vi "MeasureProcess_FGV.vi"(0 "write status":T1, 1 "action":T3(ring), 5 "ProjectAct step":T2(ring), 11 "error in":errorcluster, 12 "new element/subarray":string) -> (4 "read project name":string, 6 "read project step":string[](array[string]), 8 "step content":string[](array[string]), 10 "Table Control":string[][](table), 15 "error out":errorcluster)   [LabVIEW 2019]
uses:
  Ctrl/ProjectNameSelect.ctl
  e17d802b-cf53-46b2-bed7-7df0a5bdc549.vi
  <vilib>/JDP Science/JSONtext/Variant to JSON Text.vi
  fab65405-55d6-4226-9659-8694a5ed6800.vi
  LLB/Commonly VI/Main Glb.vi
  LLB/Commonly VI.lvlib
  <vilib>/drjdpowell/SQLite Library/SQL Connection/Execute SQL (Single String).vi
panel:
  out "element":string
  in  "Project Index":i32=3
  # "Up:0\nDown:1"
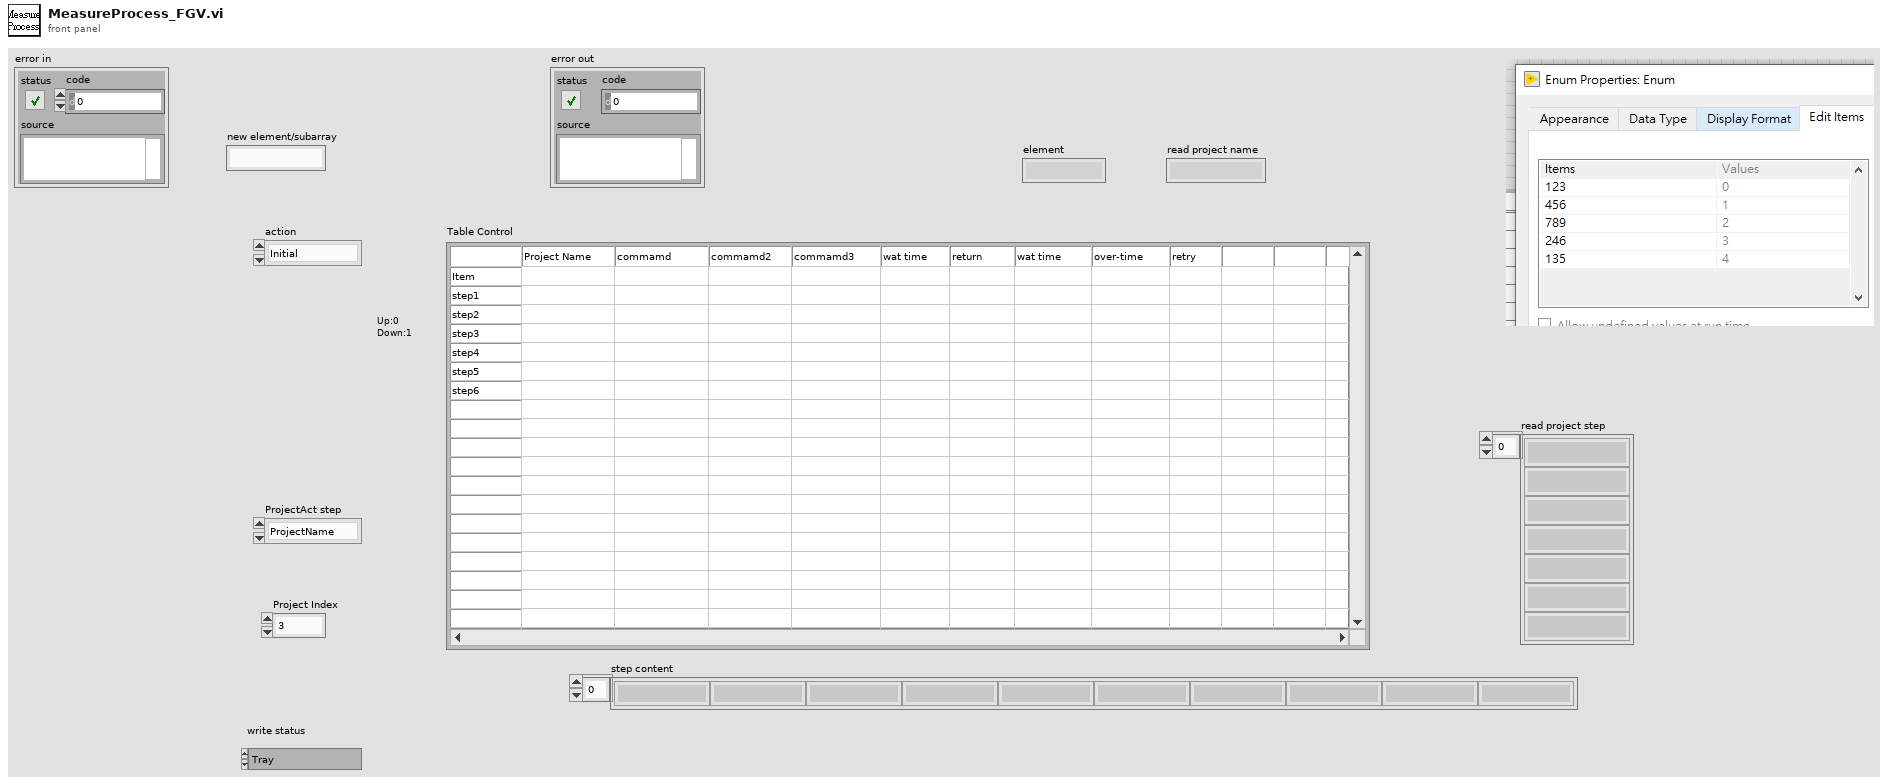
[diagram p1: front panel]
types:
  T1 = typedef "ProjectNameSelect.ctl" = enum16{"Tray", "NewItem", "NoTray", "Working", "OK"}
  T2 = enum16{"ProjectName", "Name", "Initial", "Reset", "Format", "Program1", "Program2", "Scan"}
  T3 = enum16{"Initial", "load", "read", "write", "write sn", "save"}
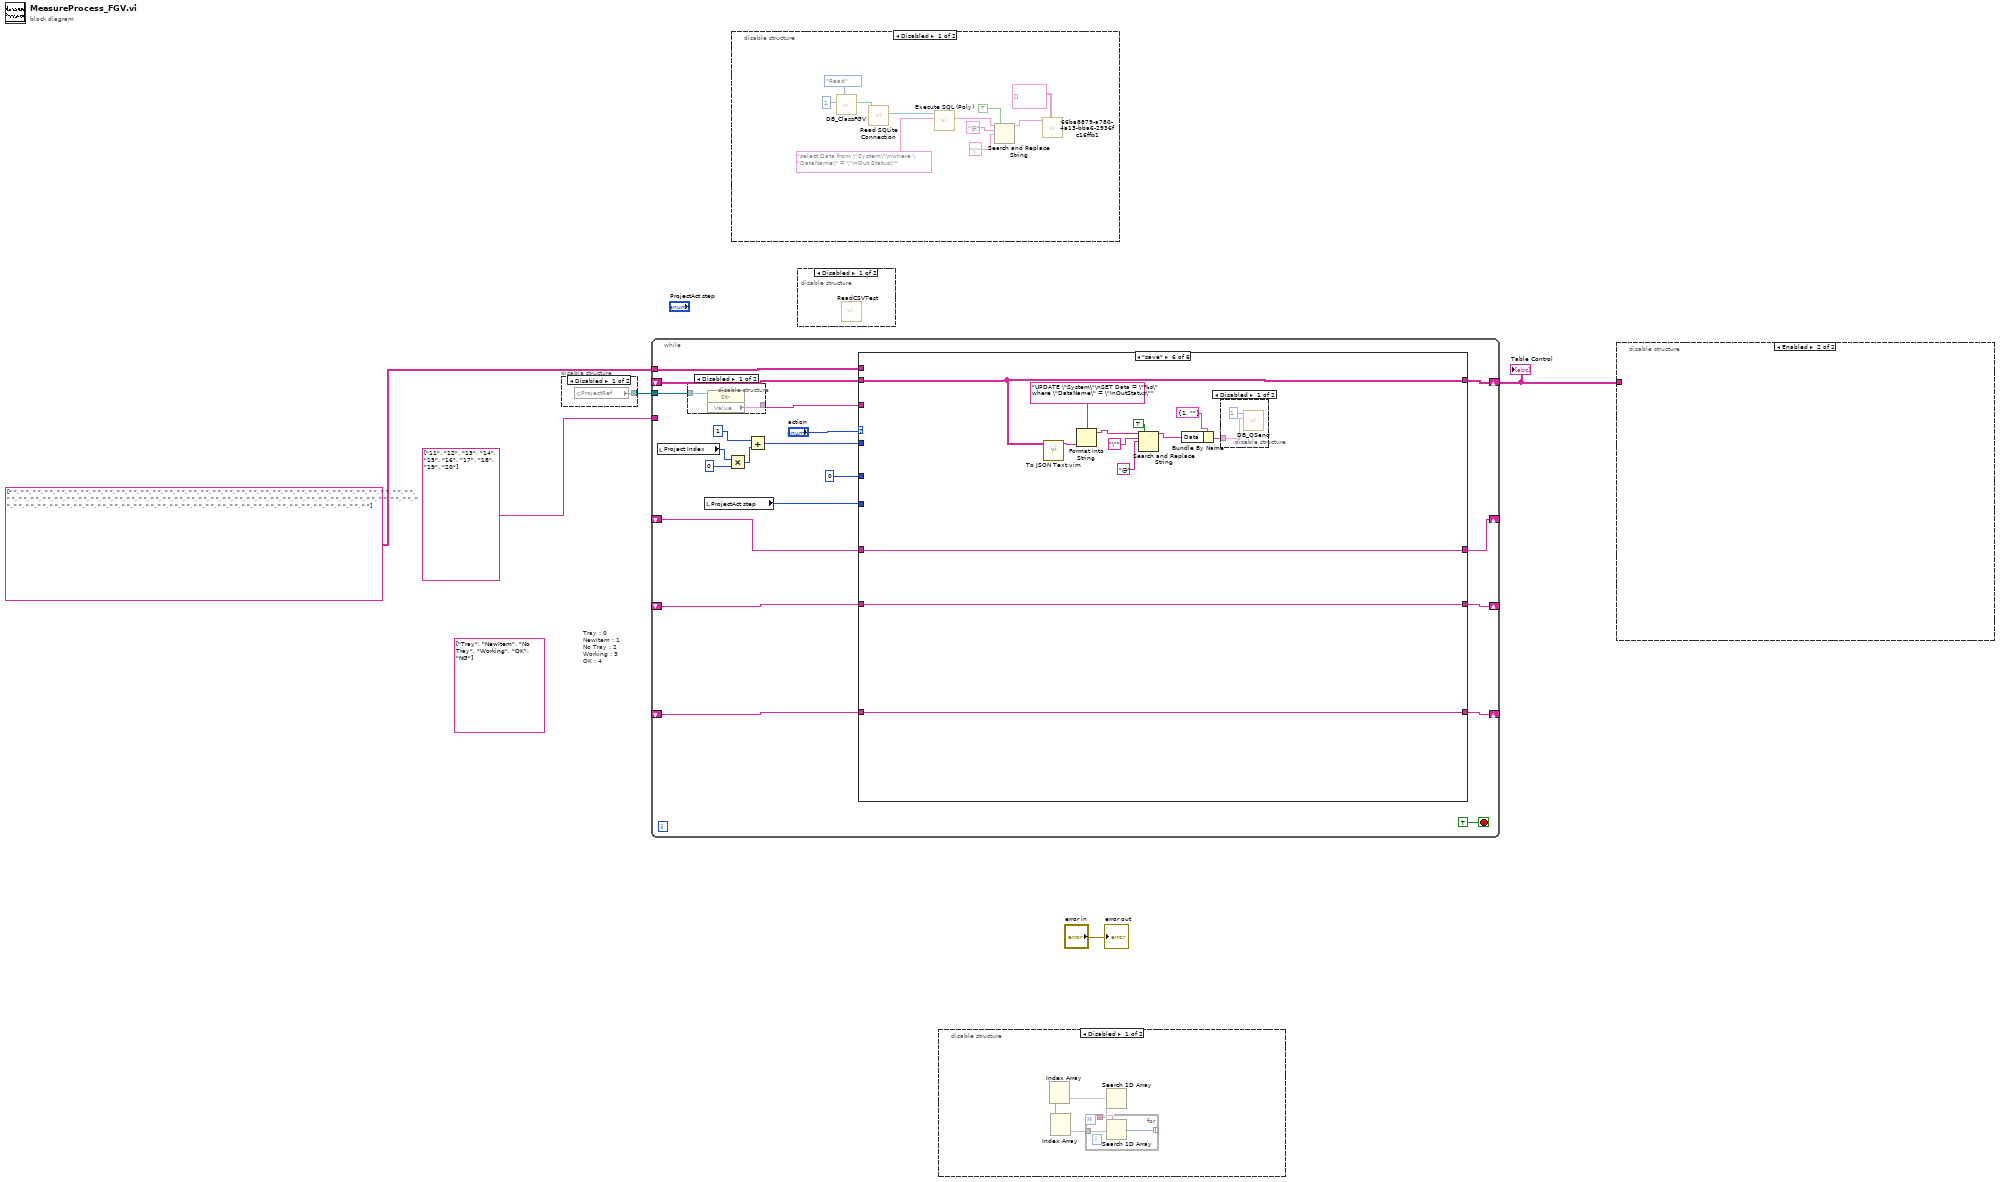
[diagram p0: block diagram]
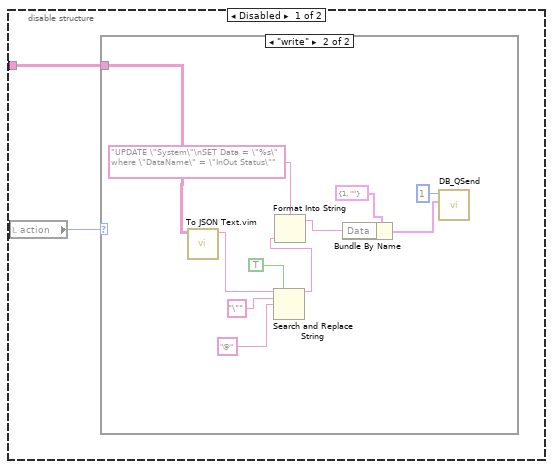
[diagram p6: hidden frame]
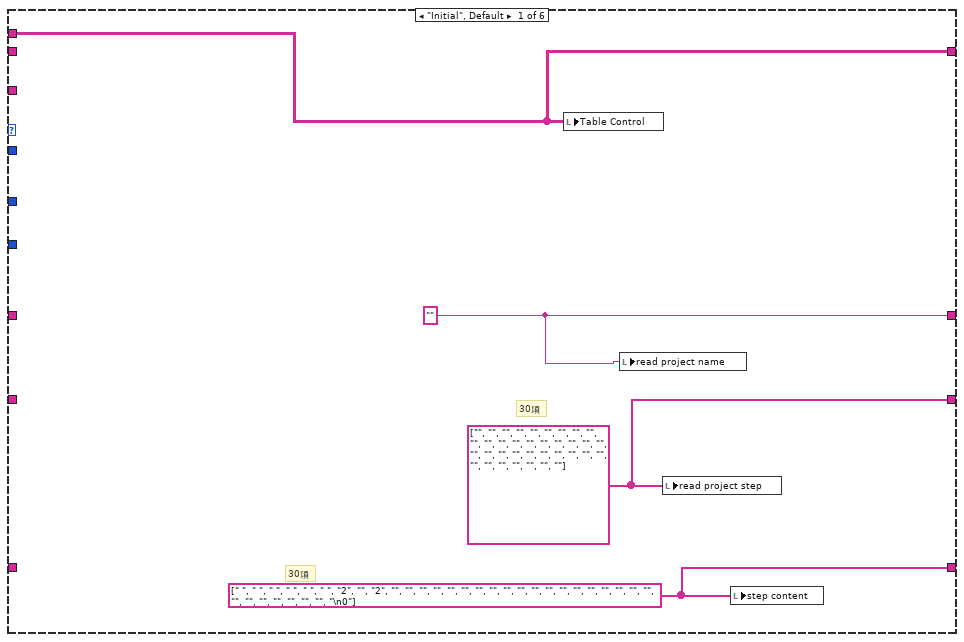
[diagram p9: hidden frame]
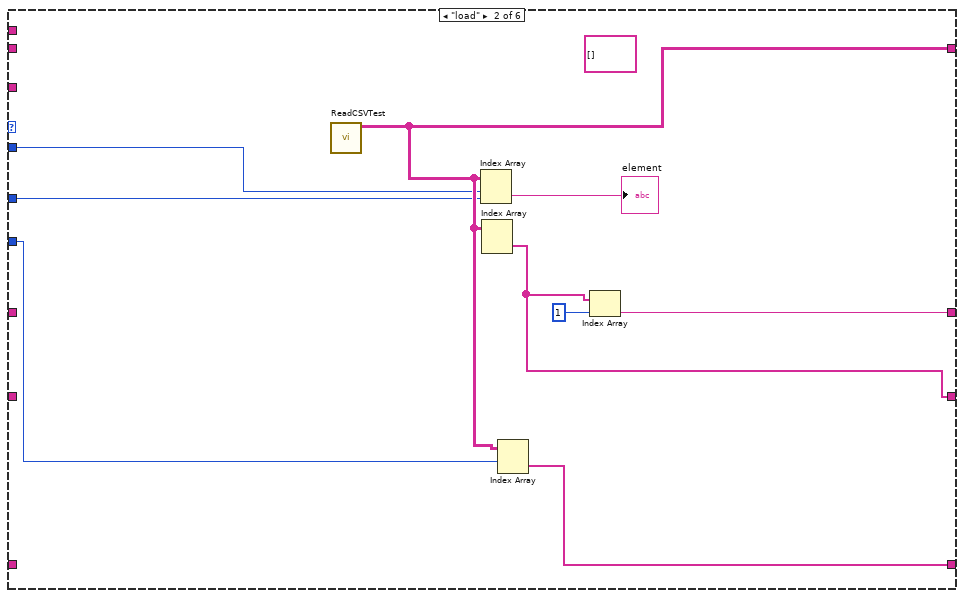
[diagram p10: hidden frame]
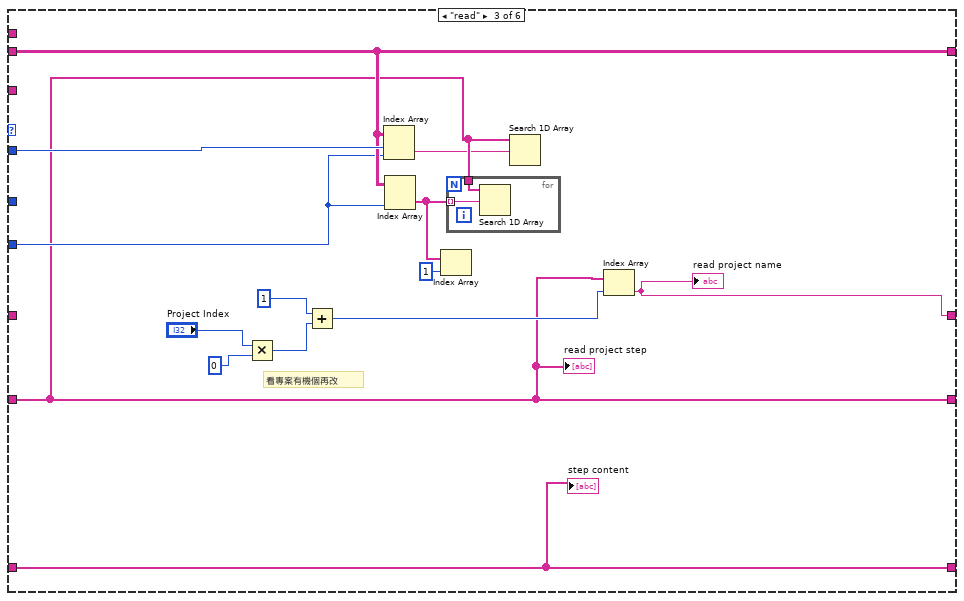
[diagram p11: hidden frame]
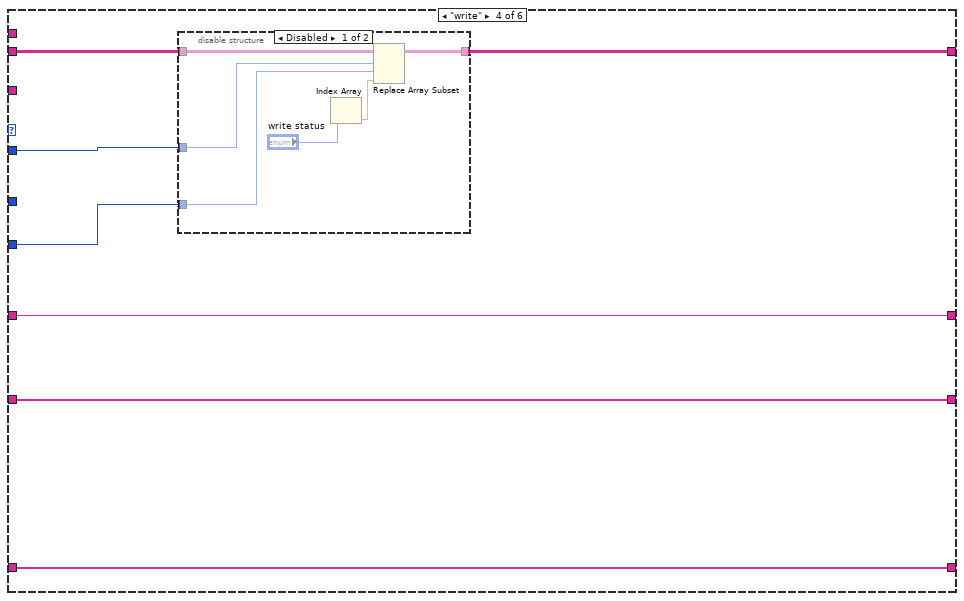
[diagram p12: hidden frame]
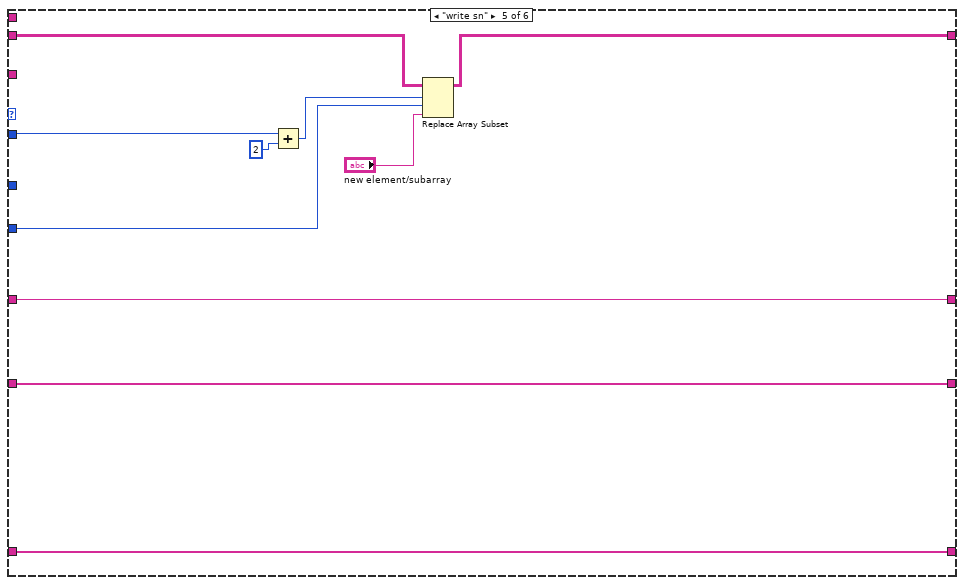
[diagram p14: hidden frame]
diagram:
  (unwired) string[] ["Tray", "NewItem", "No Tray", "Working", "OK", "NG"]
  # "Tray : 0\nNewItem : 1\nNo Tray : 2\nWorking : 3\nOK : 4"
  n1 = disable-structure shown="Disabled" {
    disable-tunnel: [w6 _] -> w2
    frame Disabled {
      n2 = global read "Main Glb.vi" "ProjectRef"() -> (w6:refnum<vi>)
    }
    frame Enabled {
    }
  }
  n3 = while {
    shift-right: [w24] -> w4
    shift-left: _ -> [w23]
    tunnel: string[] ["11", "12", "13", "14", "15", "16", "17", "18", "19", "20"] -> [_]
    shift-right: [w22] -> _
    shift-left: _ -> [w18]
    shift-right: [w21] -> _
    shift-left: _ -> [w17]
    shift-right: [w20] -> _
    shift-left: _ -> [w19]
    tunnel: w2 -> [w10]
    tunnel: string[][] [[" ", " ", " ", " ", " ", " ", " ", " ", " ", " ", " "], [" ", " ", " ", " ", " ", " ", " ", " ", " ", " ", " "], [" ", " ", " ", " ", " ", " ", " ", " ", " ", " ", " "], [" ", " ", " ", " ", " ", " ", " ", " ", " ", " ", " "], [" ", " ", " ", " ", " ", " ", " ", " ", " ", " ", " "], [" ", " ", " ", " ", " ", " ", " ", " ", " ", " ", " "], [" ", " ", " ", " ", " ", " ", " ", " ", " ", " ", " "], [" ", " ", " ", " ", " ", " ", " ", " ", " ", " ", " "], [" ", " ", " ", " ", " ", " ", " ", " ", " ", " ", " "]] -> [w7]
    stop <- TRUE stop-if-true
    n4 = local read "Project Index"() -> (w14:i32)
    n5 = disable-structure shown="Disabled" {
      disable-tunnel: w10 -> [w28 _]
      disable-tunnel: [w27 _] -> w9
      frame Disabled {
        n6 = property class="Str"(reference=w28) -> ("Value"=w27:string)  [unwired: 1 in, 2 out]
      }
      frame Enabled {
      }
    }
    n7 = local read "ProjectAct step"() -> (w16:T2)
    n8 = Multiply(x=w14, y=0) -> (x*y=w15:i32)
    n9 = Add(x=1, y=w15) -> (x+y=w11:i32)
    n10 = case shown="\"save\"" "action" {
      tunnel: [w29 w41 w54 w63 w79 w85] -> w24
      tunnel: w23 -> [_ _ w54 w64 w80 w85]
      tunnel: w16 -> [_ w33 w50 w62 w78 _]
      tunnel: w11 -> [_ w40 w55 w61 w76 _]
      tunnel: [w32 w36 w49 w60 w73 w83] -> w22
      tunnel: [w31 w37 w43 w59 w72 w82] -> w21
      tunnel: [w30 w39 w53 w58 w71 w81] -> w20
      tunnel: w19 -> [_ _ w53 w58 w71 w81]
      tunnel: w18 -> [_ _ _ w60 w73 w83]
      tunnel: w17 -> [_ _ w43 w59 w72 w82]
      tunnel: w9 -> [_ _ _ _ _ _]
      tunnel: 0 -> [_ w34 _ _ _ _]
      tunnel: w7 -> [w29 _ _ _ _ _]
      frame "Initial", Default {
        w30 = string[] [" ", " ", " ", " ", " ", " ", "2", "", "2", "", "", "", "", "", "", "", "", "", "", "", "", "", "", "", "", "", "", "", "", "", "", "", "", "", "", "\n0"] ("step content")
        w31 = string[] ["", "", "", "", "", "", "", "", "", "", "", "", "", "", "", "", "", "", "", "", "", "", "", "", "", "", "", "", "", "", "", "", "", "", "", ""] ("read project step")
        w32 = "" ("String")
        # "30項"
        # "30項"
        n11 = local write "Table Control"(w29) -> ()
        n12 = local write "read project name"(w32) -> ()
        n13 = local write "read project step"(w31) -> ()
        n14 = local write "step content"(w30) -> ()
      }
      frame "load" {
        (unwired) string[][] [] ("Table Control")
        n15 = call "ReadCSVTest.vi"() -> ("all rows"=w41:string[][])  [unwired: 11 in]
        n16 = Index Array(array=w41, index (row)=w40, index (col)=w34) -> (element=→"element":string)
        n17 = Index Array(array=w41) -> (element=w37:string[])  [unwired: 2 in]
        n18 = Index Array(array=w41, index (row)=w33) -> (element=w39:string[])  [unwired: 1 in]
        n19 = Index Array(array=w37, index=1) -> (element=w36:string)
      }
      frame "read" {
        # "看專案有機個再改"
        n20 = Multiply(x="Project Index", y=0) -> (x*y=w44:i32)
        n21 = Add(x=1, y=w44) -> (x+y=w47:i32)
        n22 = Index Array(array=w54, index (row)=w55, index (col)=w50) -> (element=w42:string)
        n23 = Index Array(array=w54, index (col)=w50) -> (element=w51:string[])  [unwired: 1 in]
        n24 = Index Array(array=w51, index=1) -> ()  [unwired: 1 out]
        n25 = for {
          tunnel: w43 -> [w57]
          tunnel: w51 -> [w56] mode=indexing
          n26 = Search 1D Array(1D array=w57, element=w56) -> ()  [unwired: 1 in, 1 out]
        }
        n27 = Search 1D Array(1D array=w43, element=w42) -> ()  [unwired: 1 in, 1 out]
        n28 = Index Array(array=w43, index=w47) -> (element=w49:string)
        "read project name" <- w49
        "read project step" <- w43
        "step content" <- w53
      }
      frame "write" {
        n29 = disable-structure shown="Disabled" {
          disable-tunnel: w64 -> [w70 _]
          disable-tunnel: [w69 _] -> w63
          disable-tunnel: w62 -> [w66 _]
          disable-tunnel: w61 -> [w65 _]
          frame Disabled {
            n30 = Index Array(index="write status") -> (element=w68)  [unwired: 1 in]
            n31 = Replace Array Subset(array=w70, new element=w68, index (row)=w65, index (col)=w66) -> (w69:string[][])
          }
          frame Enabled {
          }
        }
      }
      frame "write sn" {
        n32 = Add(x=w76, y=2) -> (x+y=w77:i32)
        n33 = Replace Array Subset(array=w80, new element="new element/subarray", index (row)=w77, index (col)=w78) -> (w79:string[][])
      }
      frame "save" {
        n34 = call "To JSON Text.vim"("Anything"=w85) -> ("<JSON>"=w91:string)  [unwired: 9 in, 1 out]
        n35 = Format Into String(format string="UPDATE \"System\"\nSET Data = \"%s\" where \"DataName\" = \"InOutStatus\"", w91) -> (resulting string=w87:string)  [unwired: 2 in, 1 out]
        n36 = Search and Replace String(replace all?=TRUE ("replace all? (F)"), input string=w87, search string="\"", replace string="@" ("replace string (\"\")")) -> (result string=w86:string)  [unwired: 4 in, 3 out]
        n37 = Bundle By Name(cluster=cluster{"Record":i32, "Data":string} {"Record"=1, "Data"=""} ("Data"), "Data"=w86) -> (w90:cluster{"Record":i32, "Data":string})
        n38 = disable-structure shown="Disabled" {
          disable-tunnel: w90 -> [w94 _]
          frame Disabled {
            n39 = call "DB_QSend.vi"("Data"=w94, "Threadindex"=1) -> ()  [unwired: 9 in, 1 out]
          }
          frame Enabled {
          }
        }
      }
    }
  }
  "Table Control" <- w4
  n40 = disable-structure shown="Disabled" {
    frame Disabled {
      n41 = call "DB_ClassFGV.vi"("Enum"=enum16{"initial", "Write", "Read"}."Read", "index"=1) -> ("DB Class out"=w98:refnum<class "DataBase.lvclass">)  [unwired: 7 in, 2 out]
      n42 = call-dynamic "Read SQLite Connection.vi"("DataBase in"=w98) -> ("SQLite.lvlib:Connection"=w99:refnum<class "Connection.lvclass">)  [unwired: 8 in, 2 out]
      n43 = call-poly <vilib>:"Execute SQL (Poly).vi"("SQL"="select Data from \"System\"\nwhere \"DataName\" = \"InOut Status\"", "SQLite Connection in"=w99) -> ("Result"=w103:string)  [unwired: 7 in, 2 out]
      n44 = Search and Replace String(replace all?=TRUE ("replace all? (F)"), input string=w103, search string="@" ("replace string (\"\")"), replace string="\"" ("search string")) -> (result string=w104:string)  [unwired: 4 in, 3 out]
      n45 = call "66ba8879-a780-4a13-bba6-2936fc16ffb1.vi"("Data Type and Default Value"=string[][] [], "JSON"=w104) -> ()  [unwired: 8 in, 2 out]
    }
    frame Enabled {
    }
  }
  n46 = disable-structure shown="Disabled" {
    frame Disabled {
      n47 = call "ReadCSVTest.vi"() -> ()  [unwired: 11 in, 1 out]
    }
    frame Enabled {
    }
  }
  n48 = disable-structure shown="Disabled" {
    frame Disabled {
      n49 = Index Array() -> (array=w109:string[][], element=w107, index (col)=w113:i32)  [unwired: 1 in]
      n50 = Index Array(array=w109, index (col)=w113) -> (element=w111)  [unwired: 1 in]
      n51 = Search 1D Array(element=w107) -> (1D array=w110:void[], index of element=w108:i32)  [unwired: 1 in]
      n52 = for {
        tunnel: w110 -> [w116]
        tunnel: w111 -> [w115]
        tunnel: [w114] -> w112 mode=indexing
        n53 = Search 1D Array(1D array=w116, element=w115) -> (index of element=w114:i32)  [unwired: 1 in]
      }
    }
    frame Enabled {
    }
  }
  n54 = disable-structure shown="Enabled" {
    disable-tunnel: w4 -> [w118 _]
    frame Disabled {
      n55 = local read "action"() -> (w117:T3)
      n56 = case shown="\"write\"" w117 {
        tunnel: w118 -> [_ w129]
        frame "Initial", Default {
        }
        frame "write" {
          n57 = call "To JSON Text.vim"("Anything"=w129) -> ("<JSON>"=w121:string)  [unwired: 9 in, 1 out]
          n58 = Search and Replace String(replace all?=TRUE ("replace all? (F)"), input string=w121, search string="\"", replace string="@" ("replace string (\"\")")) -> (result string=w120:string)  [unwired: 4 in, 3 out]
          n59 = Format Into String(format string="UPDATE \"System\"\nSET Data = \"%s\" where \"DataName\" = \"InOut Status\"", w120) -> (resulting string=w127:string)  [unwired: 2 in, 1 out]
          n60 = Bundle By Name(cluster=cluster{"Record":i32, "Data":string} {"Record"=1, "Data"=""} ("Data"), "Data"=w127) -> (w128:cluster{"Record":i32, "Data":string})
          n61 = call "DB_QSend.vi"("Data"=w128, "Threadindex"=1) -> ()  [unwired: 9 in, 1 out]
        }
      }
    }
    frame Enabled {
    }
  }
  "error out" <- "error in"
